vi "AoA Detection TX Target Signal.vi"() -> ()   [LabVIEW 2015]
doc: "Continuously generates a communication signal that starts immediately."
uses:
  <instrlib>/niUSRP/niUSRP Write Tx Data (CDB).vi
  <vilib>/measure/NI_MABase.lvlib
panel:
  out "Tx":bool
  in  "Enabled Channel":string="0"
  out "coerced gain":dbl format="%#_6f"
  in  "device name":refnum<k15>="192.168.10.7"
  in  "active antenna":string="TX1"
  in  "tone frequency":dbl=100000.0 format="%#_6p"
  out "Waveform Graph":waveform(dbl)[](graph)
  in  "waveform size":dbl=10000.0
  in  "timeout":dbl=10.0
  out "error out":errorcluster
  in  "stop":bool
  out "coerced carrier frequency":dbl format="%#_6p"
  out "coerced IQ rate":dbl format="%#_6p"
  in  "gain":dbl=30.0 format="%#_6f"
  in  "carrier frequency":dbl=900000000.0 format="%#_6p"
  in  "IQ rate":dbl=1000000.0 format="%#_6p"
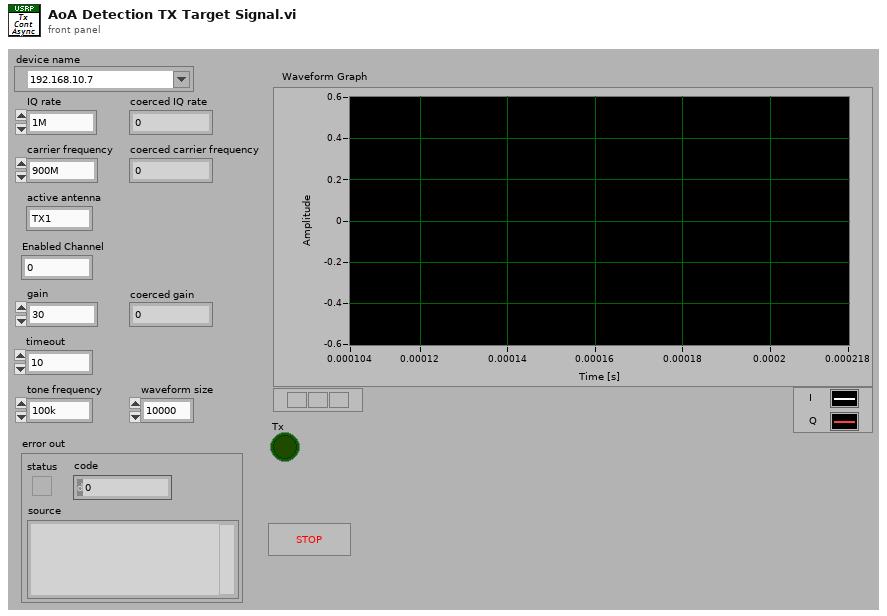
[diagram p1: front panel]
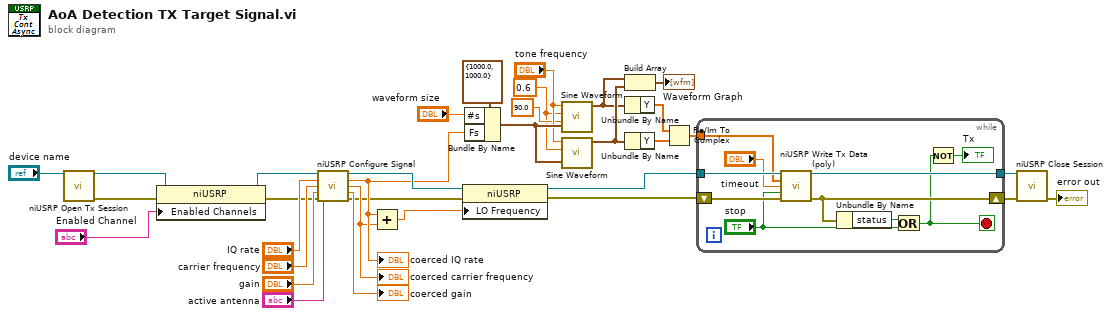
[diagram p0: block diagram]
diagram:
  w7 = 0.6 ("amplitude")
  n1 = call <instrlib>:"niUSRP Open Tx Session.vi"("device names"="device name") -> ("session handle out"=w5:refnum<k15>, "error out"=w4:errorcluster)  [unwired: 13 in]
  n2 = property class="niUSRP"(reference=w5, error in=w4, "Enabled Channels"="Enabled Channel") -> (reference out=w3:refnum<k15>, error out=w2:errorcluster)
  n3 = call <instrlib>:"niUSRP Configure Signal.vi"("session handle"=w3, "IQ rate"="IQ rate", "carrier frequency"="carrier frequency", "gain"="gain", "error in (no error)"=w2, "active antenna"="active antenna") -> ("session handle out"=w26:refnum<k15>, "coerced IQ rate"=w23:dbl, "coerced carrier frequency"=w22:dbl, "coerced gain"=→"coerced gain":dbl, "error out"=w21:errorcluster)  [unwired: 5 in]
  "coerced IQ rate" <- w23
  "coerced carrier frequency" <- w22
  n4 = Add(x=w23, y=w22) -> (x+y=w24:dbl)
  n5 = property class="niUSRP"(reference=w26, error in=w21, "LO Frequency"=w24) -> (reference out=w25:refnum<k15>, error out=w27:errorcluster)
  n6 = Bundle By Name(cluster=cluster{"Fs":dbl, "#s":dbl} {"Fs"=1000.0, "#s"=1000.0} ("sampling info"), "#s"="waveform size", "Fs"=w23) -> (w16:cluster{"Fs":dbl, "#s":dbl})
  n7 = call <vilib>:"Sine Waveform.vi"("sampling info"=w16, "phase"=90.0, "amplitude"=w7, "frequency"="tone frequency") -> ("signal out"=w13:waveform(dbl))  [unwired: 6 in, 1 out]
  n8 = call <vilib>:"Sine Waveform.vi"("sampling info"=w16, "amplitude"=w7, "frequency"="tone frequency") -> ("signal out"=w14:waveform(dbl))  [unwired: 7 in, 1 out]
  n9 = Build Array(w13, w14) -> (→"Waveform Graph":waveform(dbl)[])
  n10 = Unbundle By Name(w13) -> ("Y"=w12:dbl[])
  n11 = Unbundle By Name(w14) -> ("Y"=w11:dbl[])
  n12 = Re/Im To Complex(1:w11, 2:w12) -> (0:w9:cdb[])
  n13 = while {
    tunnel: w25 -> [w43]
    tunnel: [w40] -> w19
    shift-right: [w39] -> w18
    shift-left: w27 -> [w42]
    tunnel: w9 -> [w38]
    stop <- w34 stop-if-true
    n14 = call-poly <instrlib>:"niUSRP Write Tx Data (poly).vi"("session handle"=w43, "data"=w38, "timeout"="timeout", "end of data?"="stop", "error in (no error)"=w42) -> ("session handle out"=w40:refnum<k15>, "error out"=w39:errorcluster)  [unwired: 9 in]
    n15 = Unbundle By Name(w39) -> ("status"=w36:bool)
    n16 = Or(x=w36, y="stop") -> (x .or. y?=w34:bool)
    n17 = Not(x=w34) -> (.not. x?=→"Tx":bool)
  }
  n18 = call <instrlib>:"niUSRP Close Session.vi"("session handle"=w19, "error in (no error)"=w18) -> ("error out"=→"error out":errorcluster)  [unwired: 13 in]
